vi "Write Inlier Threshold.vi"(8 "error in (no error)":errorcluster, 10 "Inlier Threshold":dbl=0.05, 11 "Point Correspondence Params in":refnum<class "Point Correspondence Params.lvclass">) -> (0 "error out":errorcluster, 3 "Point Correspondence Params out":refnum<class "Point Correspondence Params.lvclass">)   [LabVIEW 2020, in "g_pc_toolkit.lvlib" / "Point Correspondence Params.lvclass"]
doc: "Write Inlier Threshold.\n\nSee https://pointclouds.org/documentation/classpcl_1_1registration_1_1_correspondence_rejector_sample_consensus.html for more information."
uses:
  Point Correspondence Params.lvclass
  Point Correspondence Params.lvclass/Point Correspondence Params.ctl
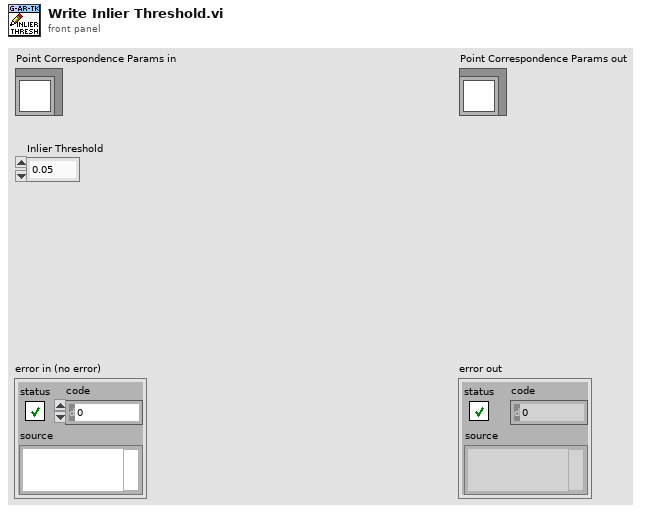
[diagram p1: front panel]
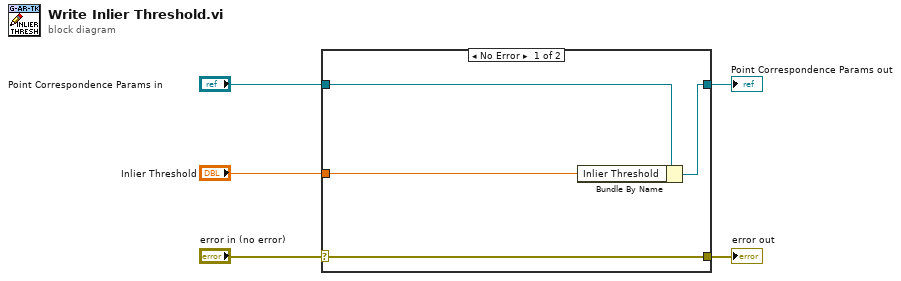
[diagram p0: block diagram]
diagram:
  n1 = case shown="No Error" "error in (no error)" {
    selector: "error in (no error)" -> [w9 w10]
    tunnel: [w9 w10] -> w4
    tunnel: [w7 w11] -> w2
    tunnel: "Point Correspondence Params in" -> [w8 w11]
    tunnel: "Inlier Threshold" -> [w6 _]
    frame No Error {
      n2 = Bundle By Name(cluster=w8, "Inlier Threshold"=w6) -> (w7:refnum<class "Point Correspondence Params.lvclass">)
    }
    frame Error {
    }
  }
  "error out" <- w4
  "Point Correspondence Params out" <- w2
